vi "Update Configuration with Existing Modules.vi"(7 "Module IDs":string[](array[string]), 8 "error in":errorcluster, 9 "Default Module Error Configuration":T1, 10 "Default Module Decimation":T5={"Decimation"=1, "Offset"=0}, 11 "Standard Engine Configuration in":refnum<class "Standard Engine Configuration.lvclass">) -> (0 "error out":errorcluster, 3 "Standard Engine Configuration out":refnum<class "Standard Engine Configuration.lvclass">)   [LabVIEW 2013, in "Standard Engine Configuration.lvclass"]
uses:
  Standard Engine Configuration.lvclass
  Module Decimation.ctl
  Module Error Configuration.ctl
  Error Actions By Category.ctl
  <vilib>/NI/Tag Bus Module Framework/runtime/error classification.ctl
  Error Actions.ctl
  Standard Engine Configuration.lvclass/Standard Engine Configuration.ctl
  Find Module Specific Config.vi
  <vilib>/Utility/error.llb/Error Cluster From Error Code.vi
  <vilib>/NI/Tag Bus Module Framework/runtime/TBM module execution interface.lvclass
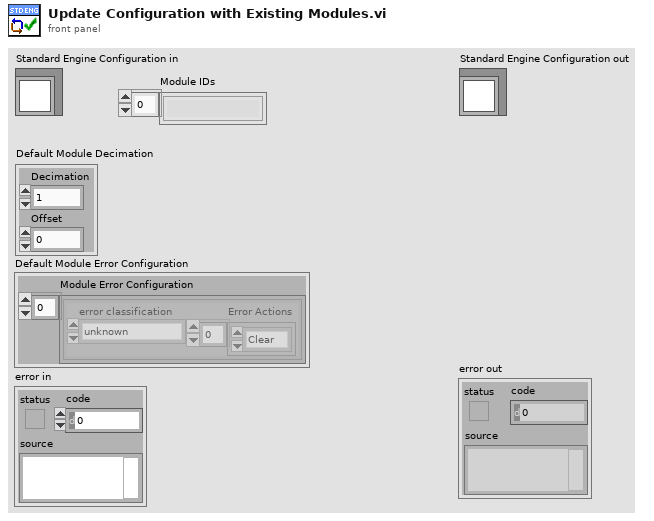
[diagram p1: front panel]
types:
  T1 = typedef "Standard Engine Configuration.lvclass/Module Error Configuration.ctl" = cluster{"Module Error Configuration":T2[]}
  T2 = typedef "Standard Engine Configuration.lvclass/Error Actions By Category.ctl" = cluster{"error classification":T3, "Error Actions":T4[]}
  T3 = typedef "TBM module execution interface.lvclass/error classification.ctl" = enum16{"unknown", "none", "trivial", "recoverable", "critical"}
  T4 = typedef "Standard Engine Configuration.lvclass/Error Actions.ctl" = enum16{"Clear", "Notify", "Stop Component", "Stop Engine", "Safe State", "Attempt Recovery"}
  T5 = typedef "Standard Engine Configuration.lvclass/Module Decimation.ctl" = cluster{"Decimation":u16, "Offset":u16}
  T6 = typedef "Standard Engine Configuration.lvclass/Module Specific Configuration.ctl" = cluster{"Module ID":string, "Module Decimation":T5, "Module Error Configuration":T1, "execution order priority":i32, "async?":bool}
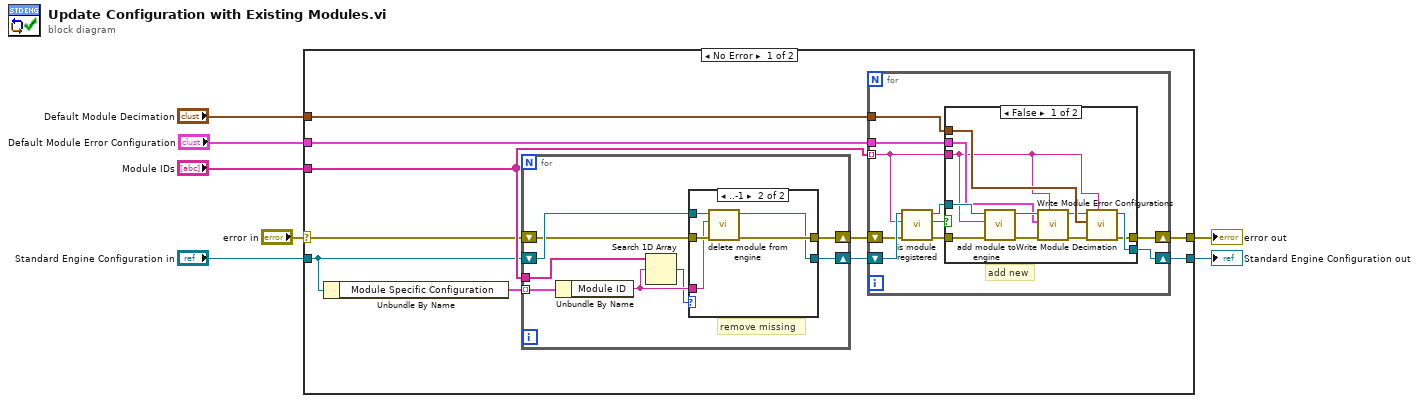
[diagram p0: block diagram]
diagram:
  n1 = case shown="No Error" "error in" {
    selector: "error in" -> [w10 w57]
    tunnel: [w14 w57] -> w6
    tunnel: [w15 w56] -> w4
    tunnel: "Standard Engine Configuration in" -> [w11 w56]
    tunnel: "Module IDs" -> [w12 _]
    tunnel: "Default Module Decimation" -> [w16 _]
    tunnel: "Default Module Error Configuration" -> [w17 _]
    frame No Error {
      n2 = Unbundle By Name(w11) -> ("Module Specific Configuration"=w13:T6[])
      n3 = for {
        tunnel: w13 -> [w25] mode=indexing
        tunnel: w12 -> [w24]
        shift-right: [w20] -> w9
        shift-left: w11 -> [w23]
        shift-right: [w21] -> w8
        shift-left: w10 -> [w22]
        # "remove missing"
        n4 = Unbundle By Name(w25) -> ("Module ID"=w19:string)
        n5 = Search 1D Array(1D array=w24, element=w19) -> (index of element=w18:i32)  [unwired: 1 in]
        n6 = case shown="..-1" w18 {
          tunnel: w23 -> [w27 w32]
          tunnel: w22 -> [w26 w31]
          tunnel: [w26 w30] -> w21
          tunnel: [w27 w29] -> w20
          tunnel: w19 -> [_ w28]
          frame 0.. {
          }
          frame ..-1 {
            n7 = call-dynamic "delete module from engine.vi"("error in"=w31, "module ID"=w28, "Standard Engine Configuration in"=w32) -> ("error out"=w30:errorcluster, "Standard Engine Configuration out"=w29:refnum<class "Standard Engine Configuration.lvclass">)  [unwired: 7 in]
          }
        }
      }
      n8 = for {
        shift-right: [w38] -> w14
        shift-left: w8 -> [w41]
        shift-right: [w39] -> w15
        shift-left: w9 -> [w42]
        tunnel: w12 -> [w36] mode=indexing
        tunnel: w17 -> [w34]
        tunnel: w16 -> [w33]
        # "add new"
        n9 = call-dynamic "is module registered.vi"("error in"=w41, "module ID"=w36, "engine configuration in"=w42) -> ("error out"=w37:errorcluster, "registered?"=w35:bool, "engine configuration out"=w40:refnum<class "Standard Engine Configuration.lvclass">)  [unwired: 6 in]
        n10 = case shown="False" w35 {
          tunnel: w40 -> [w53 w55]
          tunnel: [w45 w55] -> w39
          tunnel: [w44 w54] -> w38
          tunnel: w37 -> [w52 w54]
          tunnel: w36 -> [w43 _]
          tunnel: w34 -> [w49 _]
          tunnel: w33 -> [w48 _]
          frame False {
            n11 = call-dynamic "add module to engine.vi"("error in"=w52, "module ID"=w43, "Standard Engine Configuration in"=w53) -> ("error out"=w50:errorcluster, "Standard Engine Configuration out"=w51:refnum<class "Standard Engine Configuration.lvclass">)  [unwired: 7 in]
            n12 = call "Write Module Error Configurations.vi"("Module ID"=w43, "error in"=w50, "Module Error Configuration"=w49, "Standard Engine Repo Data in"=w51) -> ("error out"=w47:errorcluster, "Standard Engine Repo Data out"=w46:refnum<class "Standard Engine Configuration.lvclass">)  [unwired: 6 in]
            n13 = call "Write Module Decimation.vi"("Module ID"=w43, "error in"=w47, "Module Decimation"=w48, "Standard Engine Repo Data in"=w46) -> ("error out"=w44:errorcluster, "Standard Engine Repo Data out"=w45:refnum<class "Standard Engine Configuration.lvclass">)  [unwired: 6 in]
          }
          frame True {
          }
        }
      }
    }
    frame Error {
    }
  }
  "error out" <- w6
  "Standard Engine Configuration out" <- w4
